vi "Shooting Module.vi"(11 "distance\n(Meters)":dbl(slide) scale=0.0..6.0 scale format="%3d") -> (2 "Magnitude":dbl, 3 "Encoder Degrees":dbl)   [LabVIEW 2013]
panel:
  out "distance\n(Feet)":dbl(slide) scale=0.0..20.0 scale format="%3d"
  out "Shooting Range":bool
  out "RPM":i32
  out "Catapult Move\nAngle":i32
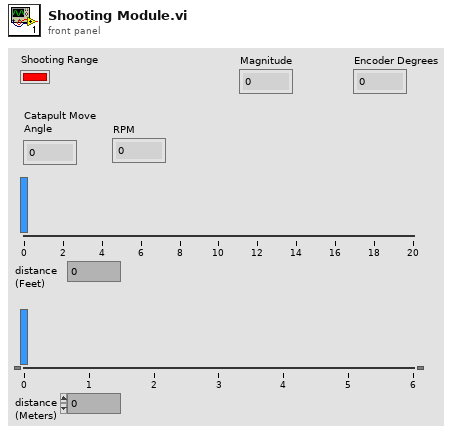
[diagram p1: front panel]
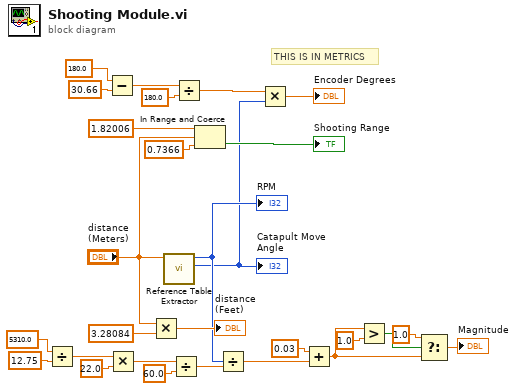
[diagram p0: block diagram]
diagram:
  # "THIS IS IN METRICS"
  n1 = Divide(x=5310.0, y=12.75) -> (x/y=w26:dbl)
  n2 = Subtract(x=180.0, y=30.66) -> (x-y=w9:dbl)
  n3 = Multiply(x=w26, y=22.0) -> (x*y=w24:dbl)
  n4 = Multiply(x="distance\n(Meters)", y=3.28084) -> (x*y=→"distance\n(Feet)":dbl)
  n5 = call "Reference Table Extractor.vi"("distance"="distance\n(Meters)") -> ("Catapult Move\nAngle"=w4:i32, "RPM"=w6:i32)  [unwired: 7 in, 2 out]
  "Catapult Move\nAngle" <- w4
  "RPM" <- w6
  n6 = Divide(x=w24, y=60.0) -> (x/y=w18:dbl)
  n7 = Divide(x=w9, y=180.0) -> (x/y=w7:dbl)
  n8 = In Range and Coerce(upper limit=1.82006, x="distance\n(Meters)", lower limit=0.7366 ("y")) -> (In Range?=→"Shooting Range":bool)  [unwired: 1 out]
  n9 = Divide(x=w6, y=w18) -> (x/y=w3:dbl)
  n10 = Multiply(x=w7, y=w4) -> (x*y=→"Encoder Degrees":dbl)
  n11 = Add(x=0.03, y=w3) -> (x+y=w2:dbl)
  n12 = Greater?(x=w2, y=1.0) -> (0:w21:bool)
  n13 = Select(t=1.0, s=w21, f=w2) -> (s? t:f=→"Magnitude":dbl)
